vi "get TextSummary.vi"(8 "error in (no error)":errorcluster, 11 "Channel in":refnum<class "Parameter.lvclass">) -> (0 "error out":errorcluster, 2 "Text Summary":string, 3 "Channel out":refnum<class "Parameter.lvclass">)   [LabVIEW 2013, in "Parameter.lvclass"]
doc: "Text Summary is the string that appears in the second column of the tree control. It summaries the state of the xceDataNode."
uses:
  Parameter.lvclass
  xCE/xceNode/xceNode.lvclass
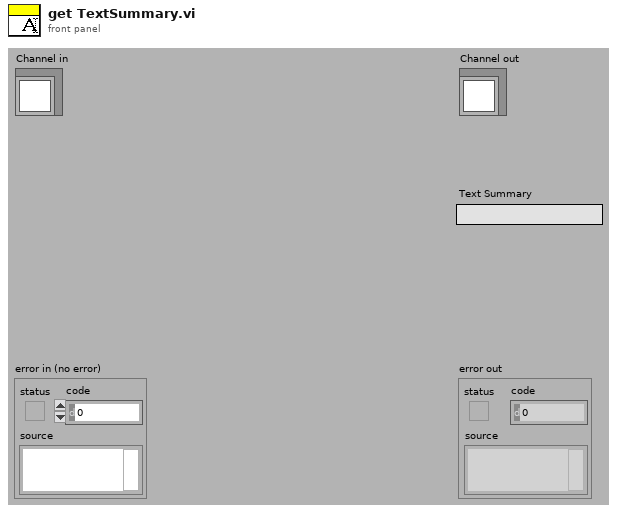
[diagram p1: front panel]
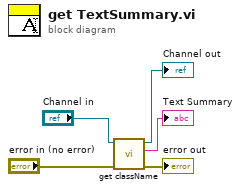
[diagram p0: block diagram]
diagram:
  n1 = call "get className.vi"("error in (no error)"="error in (no error)", "xceNode in"="Channel in") -> ("error out"=→"error out":errorcluster, "Class name"=→"Text Summary":string, "xceNode out"=→"Channel out":refnum<class "Parameter.lvclass">)  [unwired: 7 in]
